vi "adatok_mappa.vi"() -> (3 "*\\adatok mappa útvonala":path)   [LabVIEW 2014]
doc: "Az *\\adatok mappa útvonalának összeállítása."
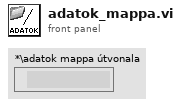
[diagram p1: front panel]
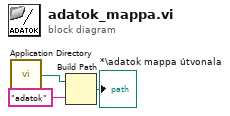
[diagram p0: block diagram]
diagram:
  n1 = call <vilib>:"Application Directory.vi"() -> ("Application Directory"=w3:path)
  n2 = Build Path(base path=w3, name or relative path="adatok") -> (appended path=→"*\\adatok mappa útvonala":path)
